vi "Variable list Tractor digital.vi"() -> (6 "Variant":variant, 10 "Array":T1[](array[typedef]))   [LabVIEW 2011]
uses:
  Measurments Handling/Fixed Digital Channel Definition.ctl
  Measurments Handling/Update frequensies.ctl
  Measurments Handling/Channel catagory Enum.ctl
  Variable List Tractor Digital.ctl
  <vilib>/Utility/VariantDataType/GetNumericInfo.vi
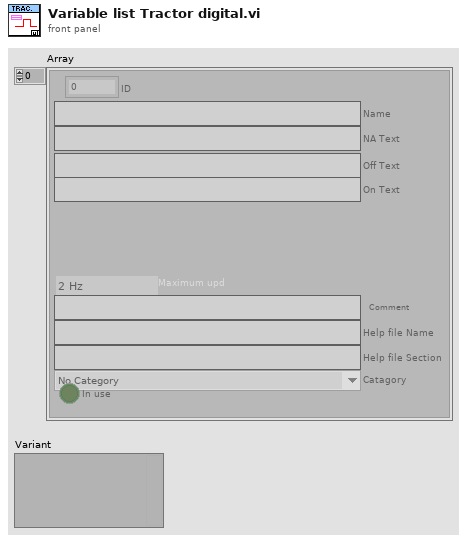
[diagram p1: front panel]
types:
  T1 = typedef "Fixed Digital Channel Definition.ctl" = cluster{"ID":u16, "Name":string, "NA Text":string, "Off Text":string, "On Text":string, "Maximum upd":T2, "Comment":string, "Help file Name":string, "Help file Section ":string, "Catagory":T3, "In use":bool}
  T2 = typedef "Update frequensies.ctl" = enum16{"2 Hz", "1 Hz", "0.1 Hz"}
  T3 = typedef "Channel catagory Enum.ctl" = enum16{"No Category", "Power", "Temperature", "Pressure"}
  T4 = typedef "Variable List Tractor Digital.ctl" = enum16{"Tractor Relay 1", "Tractor Relay 2", "Tractor Upper Tension Sub", "Tractor Lower Tension Sub", "Tractor Controller error", "Tractor Upper Tension Sub error", "Tractor Lower Tension Sub error", "Tractor Controller stopped", "Tractor Upper Tension Sub stopped", "Tractor Lower Tension Sub stopped"}
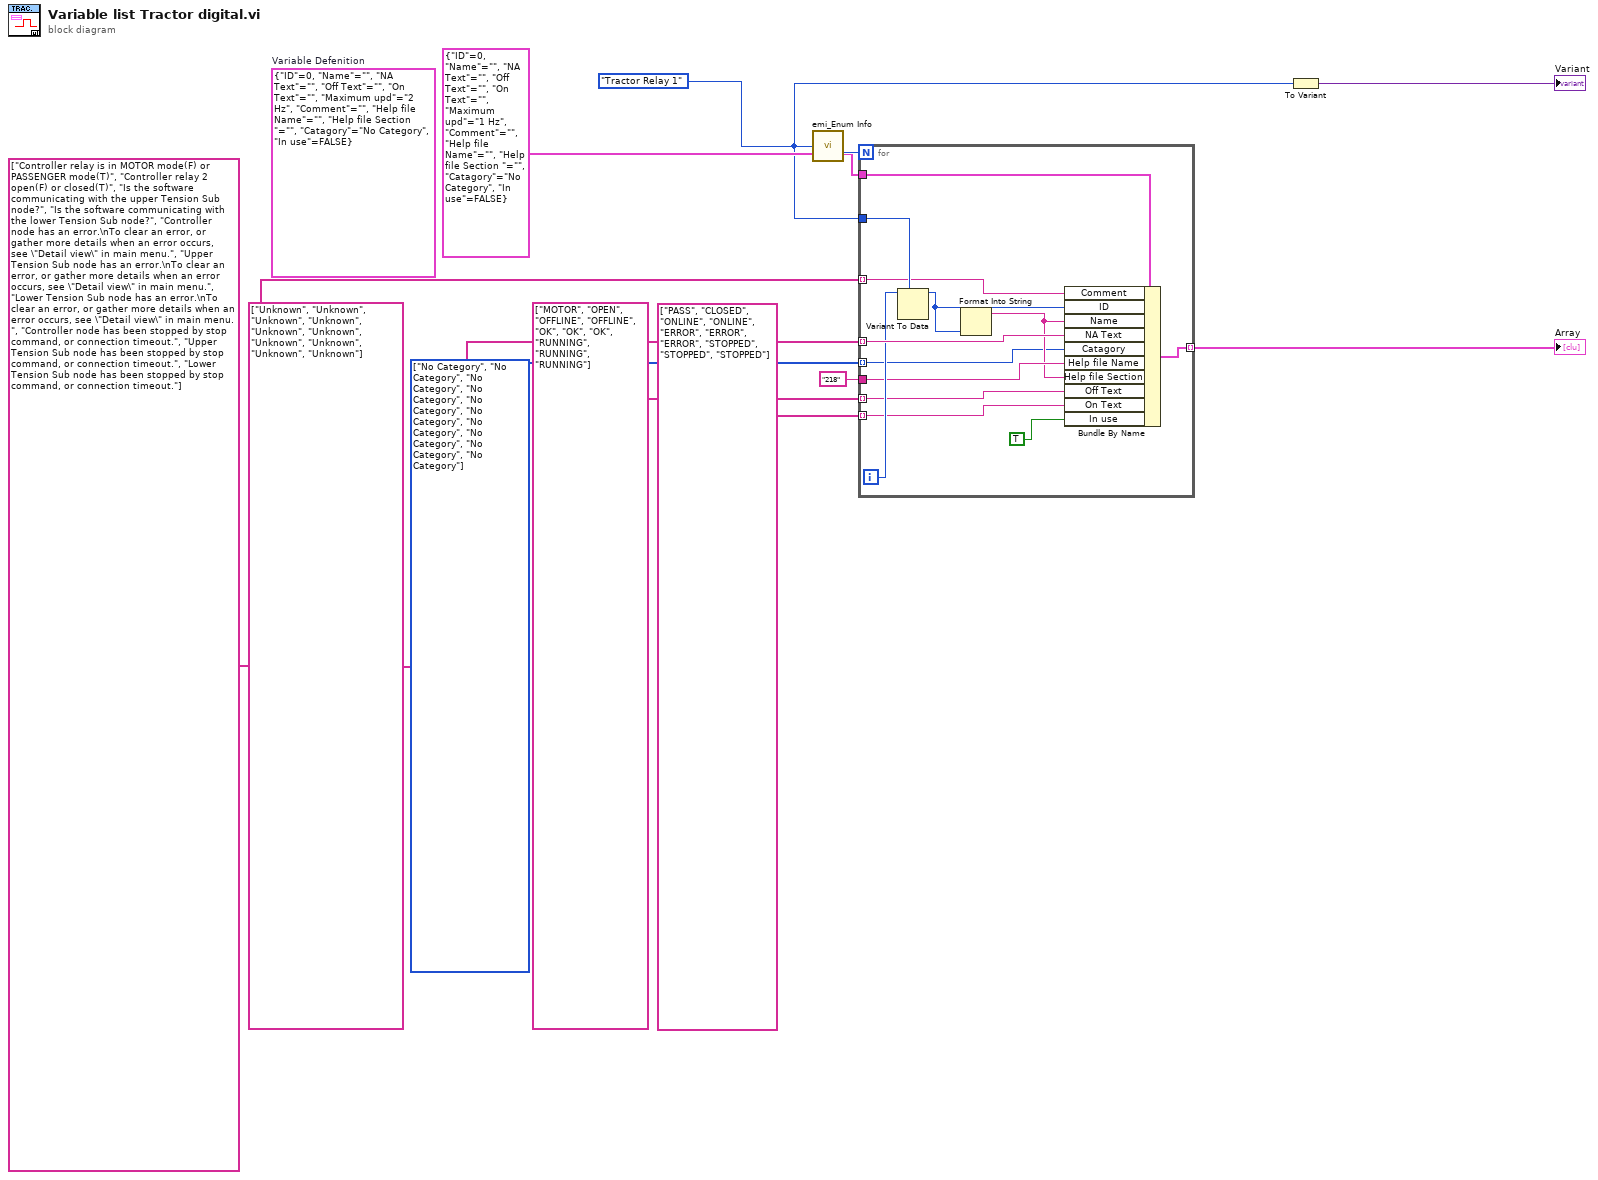
[diagram p0: block diagram]
diagram:
  w1 = Variable_List_Tractor_Digital."Tractor Relay 1" ("Action")
  (unwired) T1 {"ID"=0, "Name"="", "NA Text"="", "Off Text"="", "On Text"="", "Maximum upd"=enum."2 Hz", "Comment"="", "Help file Name"="", "Help file Section "="", "Catagory"=enum."No Category", "In use"=FALSE}  # Variable Defenition
  w6 = T3[] [enum."No Category", enum."No Category", enum."No Category", enum."No Category", enum."No Category", enum."No Category", enum."No Category", enum."No Category", enum."No Category", enum."No Category"] items=["No Category", "Power", "Temperature", "Pressure"]
  n1 = call "emi_Enum Info.vi"("Enum"=w1) -> ("Numb Elements"=w3:i32)  [unwired: 11 in, 3 out]
  n2 = for {
    N: w3 -> [_]
    tunnel: w1 -> [w24]
    tunnel: T1 {"ID"=0, "Name"="", "NA Text"="", "Off Text"="", "On Text"="", "Maximum upd"=enum."1 Hz", "Comment"="", "Help file Name"="", "Help file Section "="", "Catagory"=enum."No Category", "In use"=FALSE} ("Variable Defenition") -> [w21]
    tunnel: [w22] -> w10 mode=indexing
    tunnel: string[] ["Unknown", "Unknown", "Unknown", "Unknown", "Unknown", "Unknown", "Unknown", "Unknown", "Unknown", "Unknown"] -> [w20] mode=indexing
    tunnel: w6 -> [w16] mode=indexing
    tunnel: "218" -> [w18]
    tunnel: string[] ["MOTOR", "OPEN", "OFFLINE", "OFFLINE", "OK", "OK", "OK", "RUNNING", "RUNNING", "RUNNING"] -> [w15] mode=indexing
    tunnel: string[] ["PASS", "CLOSED", "ONLINE", "ONLINE", "ERROR", "ERROR", "ERROR", "STOPPED", "STOPPED", "STOPPED"] -> [w14] mode=indexing
    tunnel: string[] ["Controller relay is in MOTOR mode(F) or PASSENGER mode(T)", "Controller relay 2 open(F) or closed(T)", "Is the software communicating with the upper Tension Sub node?", "Is the software communicating with the lower Tension Sub node?", "Controller node has an error.\nTo clear an error, or gather more details when an error occurs, see \"Detail view\" in main menu.", "Upper Tension Sub node has an error.\nTo clear an error, or gather more details when an error occurs, see \"Detail view\" in main menu.", "Lower Tension Sub node has an error.\nTo clear an error, or gather more details when an error occurs, see \"Detail view\" in main menu.", "Controller node has been stopped by stop command, or connection timeout.", "Upper Tension Sub node has been stopped by stop command, or connection timeout.", "Lower Tension Sub node has been stopped by stop command, or connection timeout."] -> [w13] mode=indexing
    i -> [w19]
    n3 = Variant To Data(type=w24, Variant=w19) -> (data=w23:T4)  [unwired: 1 in, 1 out]
    n4 = Format Into String(w23) -> (resulting string=w17:string)  [unwired: 3 in, 1 out]
    n5 = Bundle By Name(cluster=w21, "Comment"=w13, "ID"=w23, "Name"=w17, "NA Text"=w20, "Catagory"=w16, "Help file Name"=w18, "Help file Section"=w17, "Off Text"=w15, "On Text"=w14, "In use"=TRUE) -> (w22:T1)
  }
  "Array" <- w10
  n6 = To Variant(anything=w1) -> (Variant=→"Variant":variant)
